vi "ProcessSerialData.vi"(10 "SerialResponseEvent":refnum<user-event>, 11 "String in":string) -> (3 "String out":string)   [LabVIEW 2022 SP3, in "GIS Printer.lvclass"]
uses:
  GIS Printer/GIS Printer.lvclass
panel:
  out "error out":errorcluster
  in  "error in (no error)":errorcluster
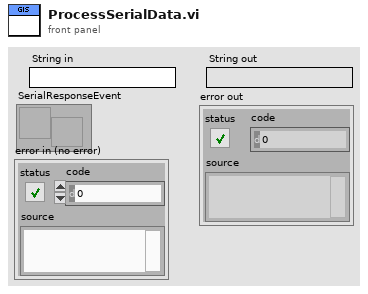
[diagram p1: front panel]
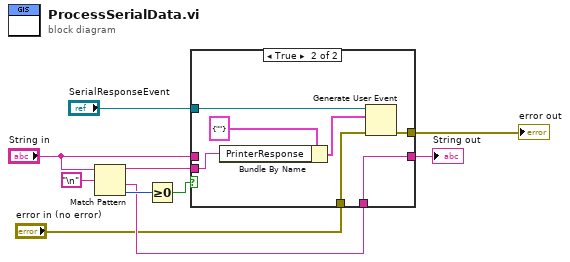
[diagram p0: block diagram]
diagram:
  n1 = Match Pattern(string="String in", regular expression="\n") -> (before substring=w8:string, after substring=w3:string, offset past match=w6:i32)  [unwired: 1 in, 1 out]
  n2 = Greater Or Equal To 0?(x=w6) -> (x >= 0?=w7:bool)
  n3 = case shown="True" w7 {
    tunnel: w8 -> [_ w16]
    tunnel: [w12 w15] -> w10
    tunnel: "String in" -> [w12 _]
    tunnel: "SerialResponseEvent" -> [_ w19]
    tunnel: w3 -> [_ w15]
    tunnel: "error in (no error)" -> [w11 w14]
    tunnel: [w11 w13] -> w1
    frame False {
    }
    frame True {
      n4 = Bundle By Name(cluster=cluster{"PrinterResponse":string} {"PrinterResponse"=""} ("event data"), "PrinterResponse"=w16) -> (w17:cluster{"PrinterResponse":string})
      n5 = Generate User Event(user event=w19, event data cluster=w17, error in=w14) -> (error out=w13:errorcluster)  [unwired: 1 in, 1 out]
    }
  }
  "String out" <- w10
  "error out" <- w1
